vi "Teleop.vi"(10 "Match Info":T1={"Autonomous Elapsed Seconds"=0.0, "TeleOp Elapsed Seconds"=0.0, "Disabled Elapsed Seconds"=0.0, "Visited Autonomous"=FALSE, "Visited TeleOp"=FALSE, "Visited Disabled"=FALSE, "Autonomous Settings"={"Autonomous Style"=enum."Independent", "VI Refnum"=refnum}}, 11 "Call Context":T2) -> ()   [LabVIEW 2012]
doc: "This VI is called for each TeleOp packet received from the DS where the robot is not disabled. It is often used to read from the joysticks and update I/O or to update setpoints for timed control loops. It should complete and return within 20 milliseconds or it may miss DS packets."
uses:
  <vilib>/Rock Robotics/WPI/DriverStation/WPI_DriverStationDerivedRobotMode.ctl
  <vilib>/Rock Robotics/WPI/DriverStation/WPI_DriverStationMatch Info.ctl
  <vilib>/Rock Robotics/WPI/Relay/WPI_RelayValue.ctl
  Robot Global Data.vi
  <vilib>/Rock Robotics/WPI/Joystick/WPI_JoystickGetSetRefNum.vi
  <vilib>/Rock Robotics/WPI/RobotDrive/WPI_RobotDriveGetSetRefNum.vi
panel:
  in  "port":u16=1140
  in  "IP address":string="10.41.43.41"
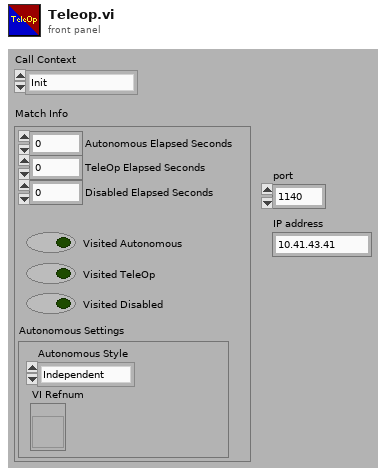
[diagram p1: front panel]
types:
  T1 = typedef "WPI_DriverStationMatch Info.ctl" = cluster{"Autonomous Elapsed Seconds":dbl, "TeleOp Elapsed Seconds":dbl, "Disabled Elapsed Seconds":dbl, "Visited Autonomous":bool, "Visited TeleOp":bool, "Visited Disabled":bool, "Autonomous Settings":cluster{"Autonomous Style":enum16{"Iterative", "Independent"}, "VI Refnum":refnum<vi>}}
  T2 = typedef "WPI_DriverStationDerivedRobotMode.ctl" = enum16{"Init", "Execute", "Stop"}
  T3 = typedef "WPI_RelayValue.ctl" = enum16{"Off", "On", "Forward", "Reverse"}
  T4 = typedef "WPI_JoystickDevRef.ctl" = cluster{"Device":T5}
  T5 = typedef "WPI_JoystickDeviceEnum.ctl" = enum16{"USB 1", "USB 2", "USB 3", "USB 4", "Kinect 1", "Kinect 2"}
  T6 = typedef "WPI_JoystickButtonState.ctl" = cluster{"Button 1":bool, "Button 2":bool, "Button 3":bool, "Button 4":bool, "Button 5":bool, "Button 6":bool, "Button 7":bool, "Button 8":bool, "Button 9":bool, "Button 10":bool, "Button 11":bool, "Button 12":bool}
  T7 = cluster{"axis 1 (x)":dbl, "axis 2 (y)":dbl, "axis 3 (throttle)":dbl, "axis 4":dbl, "axis 5":dbl, "axis 6":dbl}
  T8 = typedef "WPI_EncoderDevRef.ctl" = cluster{"DevStatus":errorcluster, "EncoderIndex":T9, "CounterIndex":T10, "DistancePerCount":dbl, "Decoding Type":T11}
  T9 = typedef "FPGA_EncoderIdx.ctl" = enum8{"Enc 0", "Enc 1", "Enc 2", "Enc 3", "Invalid"}
  T10 = typedef "FPGA_CounterCtrSystemIndex.ctl" = enum8{"Ctr 0", "Ctr 1", "Ctr 2", "Ctr 3", "Ctr 4", "Ctr 5", "Ctr 6", "Ctr 7", "Invalid"}
  T11 = typedef "WPI_EncoderType.ctl" = enum16{"1x", "2x", "4x"}
  T12 = typedef "WPI_RelayDevRef.ctl" = cluster{"DevStatus":errorcluster, "Relay Channel":T13, "Digital Module":T14, "Relay Direction":T15}
  T13 = typedef "FPGA_DIORelayChannel.ctl" = enum8{"Relay 1", "Relay 2", "Relay 3", "Relay 4", "Relay 5", "Relay 6", "Relay 7", "Relay 8", "Invalid"}
  T14 = typedef "FPGA_TypedefDigitalModule.ctl" = enum16{"Digital Module 1", "Digital Module 2"}
  T15 = typedef "WPI_RelayDirection.ctl" = enum16{"Both directions", "Forward only", "Reverse only"}
  T16 = typedef "WPI_ServoDeviceRef.ctl" = cluster{"DeviceStatus":errorcluster, "Digital Module":T14, "PWM Channel":T17, "DeadBand":T18}
  T17 = typedef "FPGA_DIOPWMChannel.ctl" = enum8{"PWM 1", "PWM 2", "PWM 3", "PWM 4", "PWM 5", "PWM 6", "PWM 7", "PWM 8", "PWM 9", "PWM 10", "Invalid"}
  T18 = typedef "WPI_PWMDeadband.ctl" = cluster{"Name":string, "maxPositivePwm":i32, "minPositivePwm":i32, "centerPwm":i32, "maxNegativePwm":i32, "minNegativePwm":i32, "angularRange":u16}
  T19 = typedef "WPI_MotorControlDeviceRef.ctl" = cluster{"DeviceStatus":errorcluster, "Type":enum16{"PWM", "CAN"}, "PWM":cluster{"Digital Module":T14, "PWM Channel":T17, "DeadBand":T18}, "CAN":cluster{"Device Number":u8, "Control Mode":T20, "Semaphore":T21, "Max Vout":dbl}, "Invert":bool, "TransformRef":T22, "InvTransformRef":T22}
  T20 = typedef "WPI_CANJaguar_ControlMode.ctl" = enum8{"Percent VBus", "Current", "Speed", "Position", "Voltage"}
  T21 = typedef "Semaphore RefNum" = refnum<k1>
  T22 = typedef "WPI_PWMTransform_ConPane.ctl" = refnum<vi>
  T23 = typedef "WPI_RobotDriveDevRef.ctl" = cluster{"DevStatus":errorcluster, "Motors[]":T19[], "Square Inputs":bool, "Max Output":dbl, "Isochronous":bool}
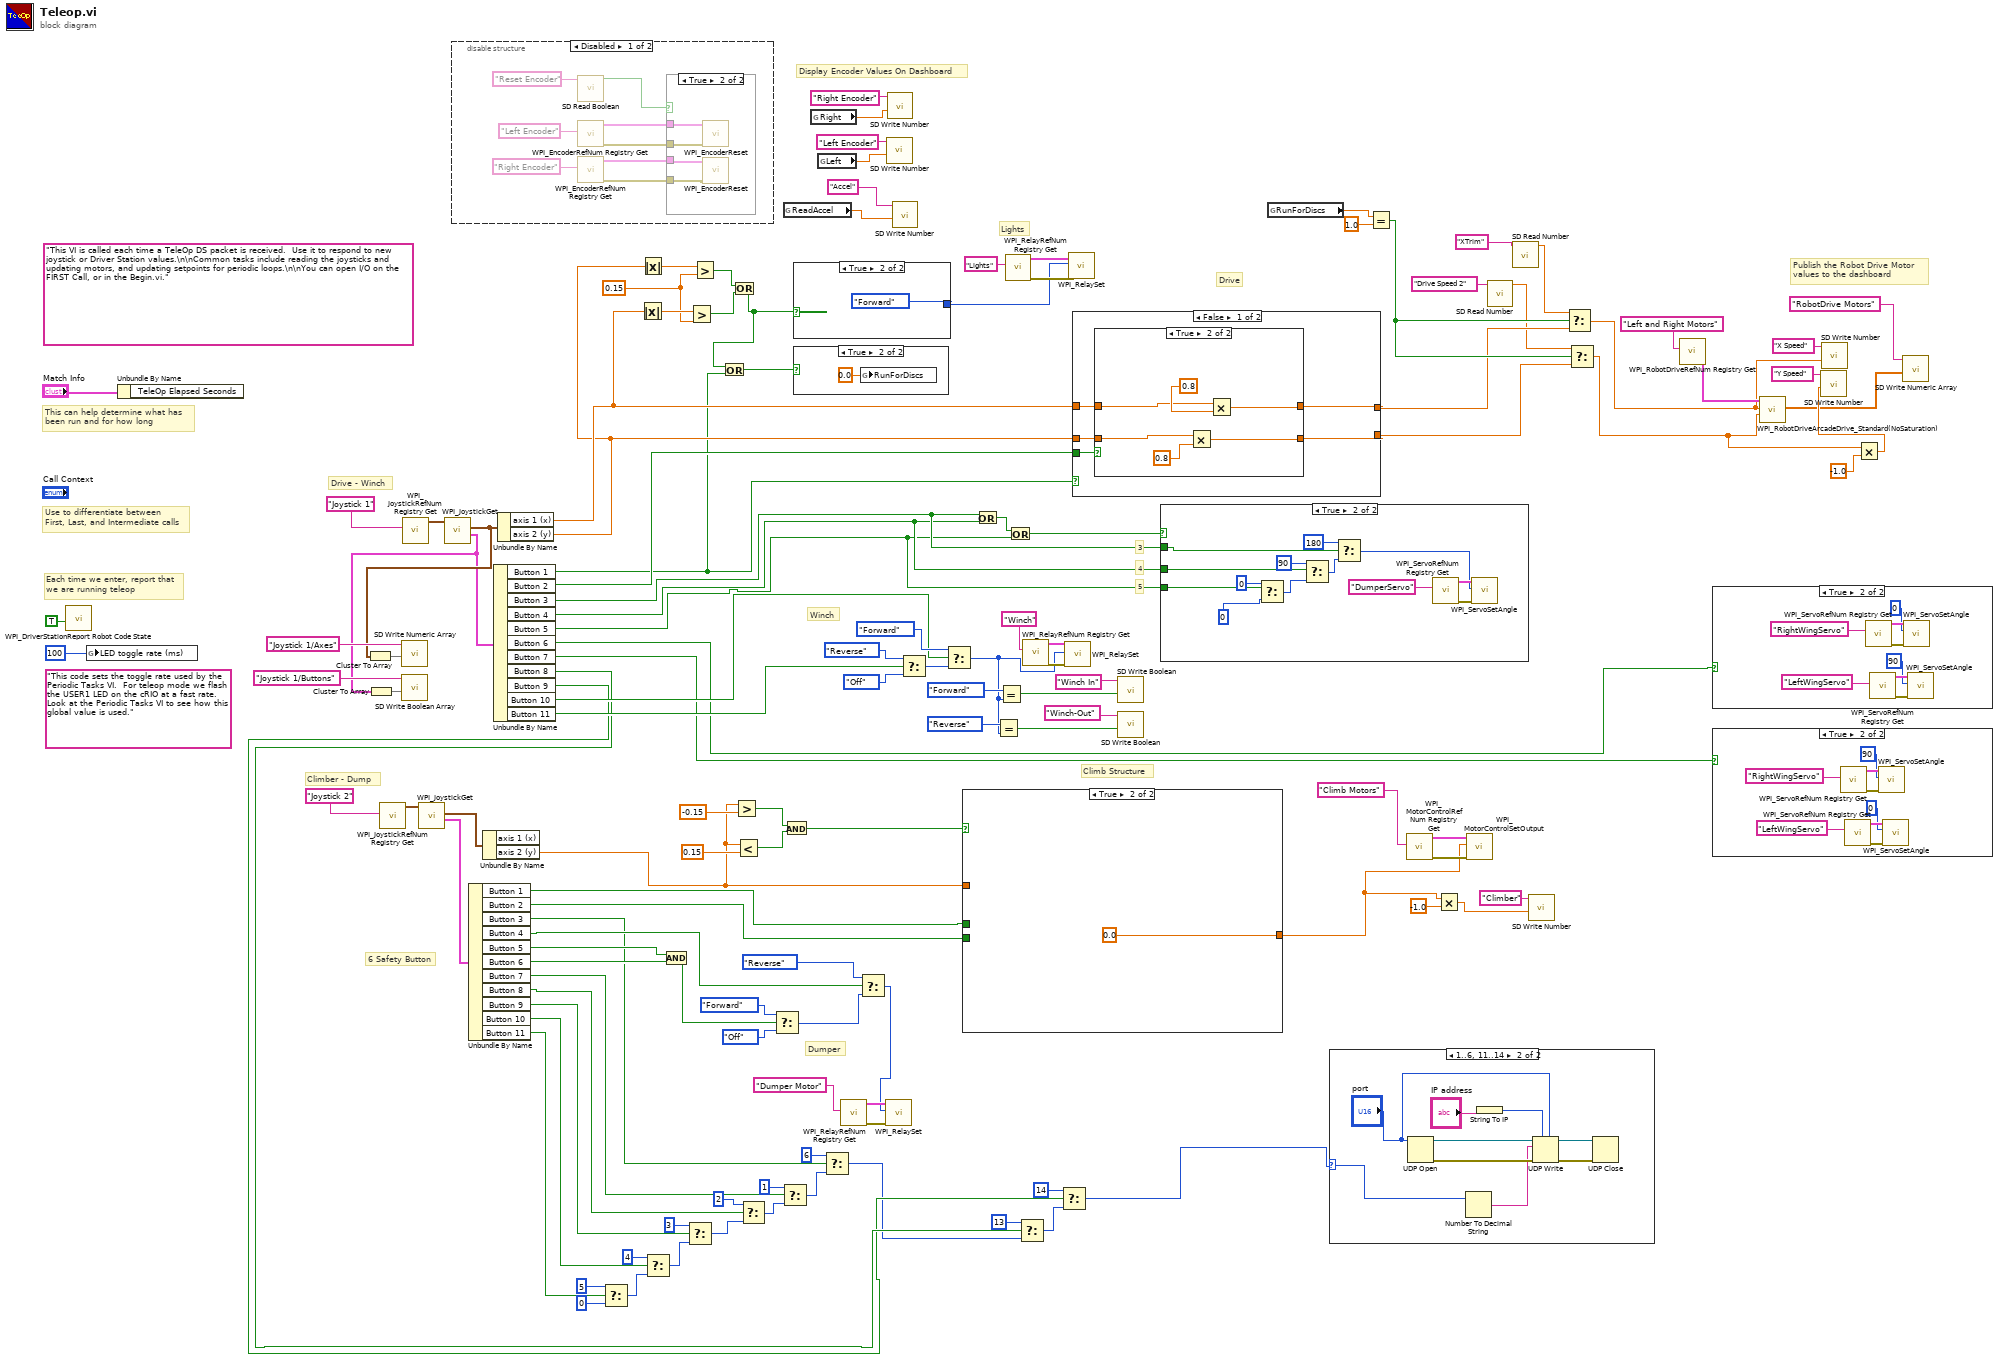
[diagram p0: block diagram]
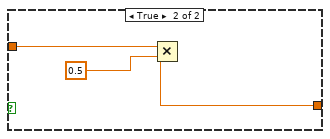
[diagram p10: hidden frame]
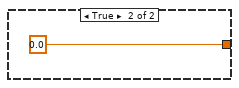
[diagram p11: hidden frame]
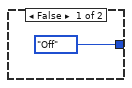
[diagram p12: hidden frame]
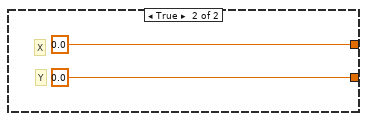
[diagram p14: hidden frame]
diagram:
  w117 = 0.15
  (unwired) "This code sets the toggle rate used by the Periodic Tasks VI.  For teleop mode we flash the USER1 LED on the cRIO at a fast rate.  Look at the Periodic Tasks VI to see how this global value is used."
  (unwired) "This VI is called each time a TeleOp DS packet is received.  Use it to respond to new joystick or Driver Station values.\n\nCommon tasks include reading the joysticks and updating motors, and updating setpoints for periodic loops.\n\nYou can open I/O on the FIRST Call, or in the Begin.vi."
  # "5"
  # "4"
  # "3"
  # "Drive - Winch"
  # "Climber - Dump"
  # "Publish the Robot Drive Motor\nvalues to the dashboard"
  # "6 Safety Button"
  # "Dumper"
  # "Climb Structure"
  # "Winch"
  # "Drive"
  # "Lights"
  # "Display Encoder Values On Dashboard"
  # "Each time we enter, report that\nwe are running teleop"
  # "Use to differentiate between\nFirst, Last, and Intermediate calls"
  # "This can help determine what has\nbeen run and for how long"
  n1 = call <vilib>:"WPI_DriverStationReport Robot Code State.vi"("TeleOp"=TRUE ("Autonomous")) -> ()  [unwired: 10 in, 1 out]
  n2 = global write "Robot Global Data.vi" "LED toggle rate (ms)"(u32 100 ("LED ms toggle rate")) -> ()
  n3 = Unbundle By Name("Match Info") -> ()  [unwired: 1 out]
  n4 = call <vilib>:"WPI_JoystickRefNum Registry Get.vi"("refnum name"="Joystick 2") -> ("JoystickDevRef"=w95:T4)  [unwired: 9 in, 1 out]
  n5 = call <vilib>:"WPI_JoystickRefNum Registry Get.vi"("refnum name"="Joystick 1") -> ("JoystickDevRef"=w120:T4)  [unwired: 1 in, 9 out]
  n6 = call <vilib>:"WPI_JoystickGet.vi"("JoystickDevRef"=w95) -> ("Buttons"=w62:T6, "Axes"=w63:T7)  [unwired: 4 in, 1 out]
  n7 = call <vilib>:"WPI_JoystickGet.vi"("JoystickDevRef"=w120) -> ("Buttons"=w54:T6, "Axes"=w55:T7)  [unwired: 1 in, 4 out]
  n8 = Cluster To Array(cluster=w55) -> (array=w57:dbl[])
  n9 = Cluster To Array(cluster=w54) -> (array=w59:bool[])
  n10 = call <vilib>:"SD Write Numeric Array.vi"("Numeric Array"=w57, "Name"="Joystick 1/Axes") -> ()  [unwired: 8 in, 2 out]
  n11 = call <vilib>:"SD Write Boolean Array.vi"("Boolean Array"=w59, "Name"="Joystick 1/Buttons") -> ()  [unwired: 8 in, 2 out]
  n12 = disable-structure shown="Disabled" {
    frame Disabled {
      n13 = call <vilib>:"SD Read Boolean.vi"("Name"="Reset Encoder") -> ("Boolean"=w132:bool)  [unwired: 8 in, 2 out]
      n14 = call <vilib>:"WPI_EncoderRefNum Registry Get.vi"("refnum name"="Left Encoder") -> ("error out"=w135:errorcluster, "EncoderDevRef"=w131:T8)  [unwired: 9 in]
      n15 = call <vilib>:"WPI_EncoderRefNum Registry Get.vi"("refnum name"="Right Encoder") -> ("error out"=w133:errorcluster, "EncoderDevRef"=w134:T8)  [unwired: 9 in]
      n16 = case shown="True" w132 {
        tunnel: w135 -> [_ w142]
        tunnel: w134 -> [_ w141]
        tunnel: w133 -> [_ w140]
        tunnel: w131 -> [_ w139]
        frame False {
        }
        frame True {
          n17 = call <vilib>:"WPI_EncoderReset.vi"("error in (no error)"=w142, "EncoderDevRef"=w139) -> ()  [unwired: 8 in, 2 out]
          n18 = call <vilib>:"WPI_EncoderReset.vi"("error in (no error)"=w140, "EncoderDevRef"=w141) -> ()  [unwired: 8 in, 2 out]
        }
      }
    }
    frame Enabled {
    }
  }
  n19 = Unbundle By Name(w62) -> ("Button 1"=w87:bool, "Button 2"=w86:bool, "Button 3"=w29:bool, "Button 4"=w53:bool, "Button 5"=w48:bool, "Button 6"=w47:bool, "Button 7"=w30:bool, "Button 8"=w31:bool, "Button 9"=w32:bool, "Button 10"=w33:bool, "Button 11"=w34:bool)
  n20 = Unbundle By Name(w63) -> ("axis 2 (y)"=w88:dbl)  [unwired: 1 out]
  n21 = Unbundle By Name(w54) -> ("Button 1"=w6:bool, "Button 2"=w112:bool, "Button 3"=w20:bool, "Button 4"=w19:bool, "Button 5"=w18:bool, "Button 6"=w2:bool, "Button 7"=w1:bool, "Button 8"=w25:bool, "Button 9"=w24:bool, "Button 10"=w97:bool, "Button 11"=w96:bool)
  n22 = Unbundle By Name(w55) -> ("axis 1 (x)"=w114:dbl, "axis 2 (y)"=w113:dbl)
  n23 = Select(t=5, s=w34, f=0) -> (s? t:f=w45:i32)
  n24 = Absolute Value(x=w114) -> (abs(x)=w118:dbl)
  n25 = Absolute Value(x=w113) -> (abs(x)=w119:dbl)
  n26 = Select(t=4, s=w33, f=w45) -> (s? t:f=w43:i32)
  n27 = And(x=w48, y=w47) -> (x .and. y?=w65:bool)
  n28 = Select(t=3, s=w32, f=w43) -> (s? t:f=w35:i32)
  n29 = Greater?(x=w118, y=w117) -> (0:w115:bool)
  n30 = Greater?(x=w119, y=w117) -> (0:w116:bool)
  n31 = Or(x=w116, y=w115) -> (x .or. y?=w5:bool)
  n32 = Or(x=w5, y=w6) -> (x .or. y?=w4:bool)
  n33 = Greater?(x=w88, y=-0.15) -> (0:w92:bool)
  n34 = Less?(x=w88, y=0.15) -> (x < y?=w93:bool)
  n35 = Select(t=2, s=w31, f=w35) -> (s? t:f=w40:i32)
  n36 = Select(t=WPI_RelayValue."Forward" ("RelayValue"), s=w65, f=WPI_RelayValue."Off" ("RelayValue")) -> (s? t:f=w66:T3)
  n37 = Select(t=1, s=w30, f=w40) -> (s? t:f=w38:i32)
  n38 = global read "Robot Global Data.vi" "ReadAccel"() -> (w123:dbl)
  n39 = And(x=w92, y=w93) -> (x .and. y?=w91:bool)
  n40 = case shown="True" w5 {
    tunnel: [WPI_RelayValue."Off" ("RelayValue") WPI_RelayValue."Forward" ("RelayValue")] -> w49
    frame False {
    }
    frame True {
    }
  }
  n41 = case shown="True" w4 {
    frame False {
    }
    frame True {
      n42 = global write "Robot Global Data.vi" "RunForDiscs"(0.0 ("RunForDiscs")) -> ()
    }
  }
  n43 = global read "Robot Global Data.vi" "Right"() -> (w125:dbl)
  n44 = global read "Robot Global Data.vi" "Left"() -> (w124:dbl)
  n45 = Select(t=6, s=w29, f=w38) -> (s? t:f=w3:i32)
  n46 = call <vilib>:"WPI_RelayRefNum Registry Get.vi"("refnum name"="Dumper Motor") -> ("error out"=w72:errorcluster, "RelayDevRef"=w71:T12)  [unwired: 9 in]
  n47 = Select(t=WPI_RelayValue."Reverse" ("RelayValue"), s=w53, f=w66) -> (s? t:f=w68:T3)
  n48 = call <vilib>:"WPI_RelaySet.vi"("error in (no error)"=w72, "RelayValue"=w68, "RelayDevRef"=w71) -> ()  [unwired: 7 in, 2 out]
  n49 = call <vilib>:"SD Write Number.vi"("Numeric"=w124, "Name"="Left Encoder") -> ()  [unwired: 8 in, 2 out]
  n50 = call <vilib>:"SD Write Number.vi"("Numeric"=w125, "Name"="Right Encoder") -> ()  [unwired: 8 in, 2 out]
  n51 = call <vilib>:"SD Write Number.vi"("Numeric"=w123, "Name"="Accel" ("refnum name")) -> ()  [unwired: 8 in, 2 out]
  n52 = Select(t=WPI_RelayValue."Reverse" ("RelayValue"), s=w96, f=WPI_RelayValue."Off" ("RelayValue")) -> (s? t:f=w111:T3)
  n53 = Select(t=WPI_RelayValue."Forward" ("RelayValue"), s=w97, f=w111) -> (s? t:f=w100:T3)
  n54 = case shown="True" w91 {
    tunnel: w87 -> [w149 _]
    tunnel: w86 -> [w148 _]
    tunnel: w88 -> [w147 _]
    tunnel: [w146 0.0 ("Output")] -> w79
    frame False {
      n55 = case shown="False" w149 {
        tunnel: w148 -> [w152 _]
        tunnel: w147 -> [w151 _]
        tunnel: [w150 0.0 ("Output")] -> w146
        frame False {
          n56 = case shown="False" w152 {
            tunnel: w151 -> [w153 w155]
            tunnel: [w153 w154] -> w150
            frame False {
            }
            frame True {
              n57 = Multiply(x=w155, y=0.5) -> (x*y=w154:dbl)
            }
          }
        }
        frame True {
        }
      }
    }
    frame True {
    }
  }
  n58 = Or(x=w20, y=w19) -> (x .or. y?=w22:bool)
  n59 = Equal?(x=WPI_RelayValue."Reverse" ("RelayValue"), y=w100) -> (x = y?=w99:bool)
  n60 = Equal?(x=WPI_RelayValue."Forward" ("RelayValue"), y=w100) -> (x = y?=w98:bool)
  n61 = call <vilib>:"WPI_RelayRefNum Registry Get.vi"("refnum name"="Lights") -> ("error out"=w50:errorcluster, "RelayDevRef"=w51:T12)  [unwired: 9 in]
  n62 = Or(x=w22, y=w18) -> (x .or. y?=w21:bool)
  n63 = Select(t=13, s=w25, f=w3) -> (s? t:f=w27:i32)
  n64 = call <vilib>:"WPI_RelayRefNum Registry Get.vi"("refnum name"="Winch") -> ("error out"=w105:errorcluster, "RelayDevRef"=w106:T12)  [unwired: 9 in]
  n65 = Select(t=14, s=w24, f=w27) -> (s? t:f=w23:i32)
  n66 = call <vilib>:"WPI_RelaySet.vi"("error in (no error)"=w105, "RelayValue"=w100, "RelayDevRef"=w106) -> ()  [unwired: 7 in, 2 out]
  n67 = call <vilib>:"WPI_RelaySet.vi"("error in (no error)"=w50, "RelayValue"=w49, "RelayDevRef"=w51) -> ()  [unwired: 7 in, 2 out]
  n68 = case shown="False" w6 {
    tunnel: w114 -> [w163 _]
    tunnel: w113 -> [w162 _]
    tunnel: w112 -> [w161 _]
    tunnel: [w160 0.0] -> w14
    tunnel: [w159 0.0] -> w13
    frame False {
      n69 = case shown="True" w161 {
        tunnel: w163 -> [w165 w168]
        tunnel: w162 -> [w164 w171]
        tunnel: [w165 w167] -> w160
        tunnel: [w164 w166] -> w159
        frame False {
        }
        frame True {
          n70 = Multiply(x=w171, y=0.8) -> (x*y=w166:dbl)
          n71 = Multiply(x=w168, y=0.8) -> (x*y=w167:dbl)
        }
      }
    }
    frame True {
      # "Y"
      # "X"
    }
  }
  n72 = call <vilib>:"SD Write Boolean.vi"("Boolean"=w98, "Name"="Winch In") -> ()  [unwired: 8 in, 2 out]
  n73 = call <vilib>:"SD Write Boolean.vi"("Boolean"=w99, "Name"="Winch-Out") -> ()  [unwired: 8 in, 2 out]
  n74 = case shown="True" w21 {
    tunnel: w20 -> [_ w178]
    tunnel: w19 -> [_ w179]
    tunnel: w18 -> [_ w182]
    frame False {
    }
    frame True {
      n75 = Select(t=0, s=w182, f=0 ("Angle")) -> (s? t:f=w181:i32)
      n76 = Select(t=90, s=w179, f=w181) -> (s? t:f=w180:i32)
      n77 = Select(t=180, s=w178, f=w180) -> (s? t:f=w174:i32)
      n78 = call <vilib>:"WPI_ServoRefNum Registry Get.vi"("refnum name"="DumperServo") -> ("error out"=w186:errorcluster, "ServoDeviceRef"=w185:T16)  [unwired: 9 in]
      n79 = call <vilib>:"WPI_ServoSetAngle.vi"("error in (no error)"=w186, "Angle"=w174, "ServoDeviceRef"=w185) -> ()  [unwired: 7 in, 2 out]
    }
  }
  n80 = global read "Robot Global Data.vi" "RunForDiscs"() -> (w17:dbl)
  n81 = case shown="1..6, 11..14" w23 {
    selector: w23 -> [_ w187]
    frame 0, Default {
    }
    frame 1..6, 11..14 {
      n82 = UDP Open(11:"port") -> (port=w190:refnum<k16>, 0:w193:errorcluster)  [unwired: 4 in, 1 out]
      n83 = Number To Decimal String(number=w187) -> (decimal integer string=w188:string)  [unwired: 1 in]
      n84 = String To IP(1:"IP address") -> (0:w194:u32)
      n85 = UDP Write(address=w194, port or service name="port", connection ID=w190, data in=w188, 8:w193) -> (error out=w192:errorcluster, 3:w189:refnum<k16>)  [unwired: 1 in]
      n86 = UDP Close(connection ID=w189, 8:w192) -> ()  [unwired: 2 out]
    }
  }
  n87 = Equal?(x=w17, y=1.0) -> (x = y?=w15:bool)
  n88 = call <vilib>:"WPI_MotorControlRefNum Registry Get.vi"("refnum name"="Climb Motors") -> ("error out"=w84:errorcluster, "MotorControlDevRef"=w85:T19)  [unwired: 9 in]
  n89 = Multiply(x=w79, y=-1.0) -> (x*y=w80:dbl)
  n90 = call <vilib>:"WPI_MotorControlSetOutput.vi"("error in (no error)"=w84, "Output"=w79, "MotorControlDevRef"=w85) -> ()  [unwired: 6 in, 3 out]
  n91 = call <vilib>:"SD Read Number.vi"("Name"="Drive Speed 2") -> ("Numeric"=w9:dbl)  [unwired: 8 in, 2 out]
  n92 = call <vilib>:"SD Read Number.vi"("Name"="XTrim") -> ("Numeric"=w7:dbl)  [unwired: 8 in, 2 out]
  n93 = call <vilib>:"SD Write Number.vi"("Numeric"=w80, "Name"="Climber") -> ()  [unwired: 8 in, 2 out]
  n94 = Select(t=w7, s=w15, f=w14) -> (s? t:f=w11:dbl)
  n95 = Select(t=w9, s=w15, f=w13) -> (s? t:f=w12:dbl)
  n96 = call <vilib>:"WPI_RobotDriveRefNum Registry Get.vi"("refnum name"="Left and Right Motors") -> ("RobotDriveDevRef"=w78:T23)  [unwired: 1 in, 9 out]
  n97 = case shown="True" w2 {
    frame False {
    }
    frame True {
      n98 = call <vilib>:"WPI_ServoRefNum Registry Get.vi"("refnum name"="RightWingServo") -> ("error out"=w203:errorcluster, "ServoDeviceRef"=w202:T16)  [unwired: 9 in]
      n99 = call <vilib>:"WPI_ServoRefNum Registry Get.vi"("refnum name"="LeftWingServo") -> ("error out"=w200:errorcluster, "ServoDeviceRef"=w199:T16)  [unwired: 9 in]
      n100 = call <vilib>:"WPI_ServoSetAngle.vi"("error in (no error)"=w203, "Angle"=0, "ServoDeviceRef"=w202) -> ()  [unwired: 7 in, 2 out]
      n101 = call <vilib>:"WPI_ServoSetAngle.vi"("error in (no error)"=w200, "Angle"=90, "ServoDeviceRef"=w199) -> ()  [unwired: 7 in, 2 out]
    }
  }
  n102 = case shown="True" w1 {
    frame False {
    }
    frame True {
      n103 = call <vilib>:"WPI_ServoRefNum Registry Get.vi"("refnum name"="RightWingServo") -> ("error out"=w211:errorcluster, "ServoDeviceRef"=w210:T16)  [unwired: 9 in]
      n104 = call <vilib>:"WPI_ServoRefNum Registry Get.vi"("refnum name"="LeftWingServo") -> ("error out"=w208:errorcluster, "ServoDeviceRef"=w207:T16)  [unwired: 9 in]
      n105 = call <vilib>:"WPI_ServoSetAngle.vi"("error in (no error)"=w211, "Angle"=90, "ServoDeviceRef"=w210) -> ()  [unwired: 7 in, 2 out]
      n106 = call <vilib>:"WPI_ServoSetAngle.vi"("error in (no error)"=w208, "Angle"=0, "ServoDeviceRef"=w207) -> ()  [unwired: 7 in, 2 out]
    }
  }
  n107 = call <vilib>:"WPI_RobotDriveArcadeDrive_Standard(NoSaturation).vi"("Y axis value"=w12, "X axis value"=w11, "RobotDriveDevRef"=w78) -> ("Motor Values"=w60:dbl[])  [unwired: 1 in, 7 out]
  n108 = call <vilib>:"SD Write Number.vi"("Numeric"=w11, "Name"="X Speed") -> ()  [unwired: 8 in, 2 out]
  n109 = Multiply(x=w12, y=-1.0) -> (x*y=w73:dbl)
  n110 = call <vilib>:"SD Write Number.vi"("Numeric"=w73, "Name"="Y Speed") -> ()  [unwired: 8 in, 2 out]
  n111 = call <vilib>:"SD Write Numeric Array.vi"("Numeric Array"=w60, "Name"="RobotDrive Motors") -> ()  [unwired: 8 in, 2 out]
